vi "IS Close Connection.vi"(8 "error in (no error)":errorcluster, 11 "IS Session In":T1) -> (0 "error out":errorcluster)   [LabVIEW 2017]
uses:
  Custom Data Types/IS Session.ctl
  <vilib>/httpClient/ClientHandle.ctl
  <vilib>/httpClient/LabVIEWHTTPClient.lvlib
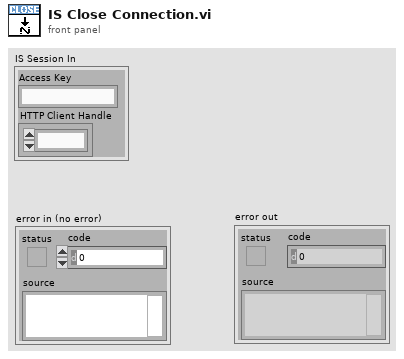
[diagram p1: front panel]
types:
  T1 = typedef "IS Session.ctl" = cluster{"Access Key":string, "HTTP Client Handle":T2}
  T2 = typedef "LabVIEWHTTPClient.lvlib/ClientHandle.ctl" = refnum<k1>
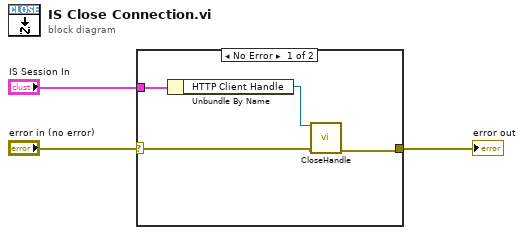
[diagram p0: block diagram]
diagram:
  n1 = case shown="No Error" "error in (no error)" {
    selector: "error in (no error)" -> [w5 w8]
    tunnel: [w4 w8] -> w3
    tunnel: "IS Session In" -> [w7 _]
    frame No Error {
      n2 = Unbundle By Name(w7) -> ("HTTP Client Handle"=w6:T2)
      n3 = call <vilib>:"CloseHandle.vi"("client handle"=w6, "error in (no error)"=w5) -> ("error out"=w4:errorcluster)  [unwired: 13 in]
    }
    frame Error {
    }
  }
  "error out" <- w3
